vi "SBE45通讯参数 (子VI).vi"() -> (0 "错误输出":errorcluster, 1 "Salinity":string, 2 "Conductivity":string, 3 "Temperature":string)   [LabVIEW 2016]
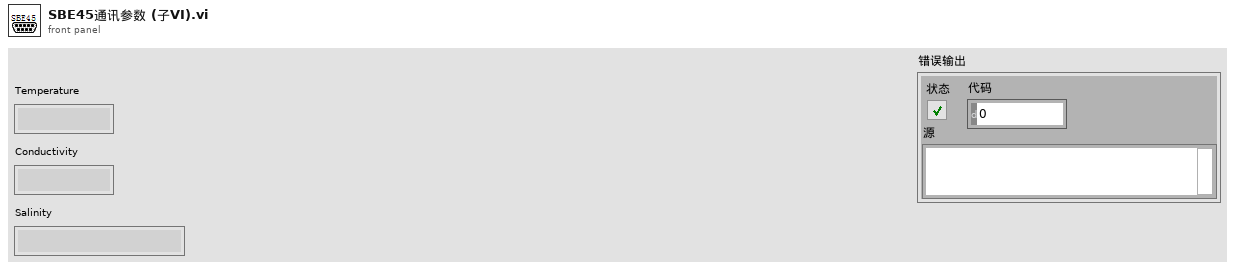
[diagram p1: front panel]
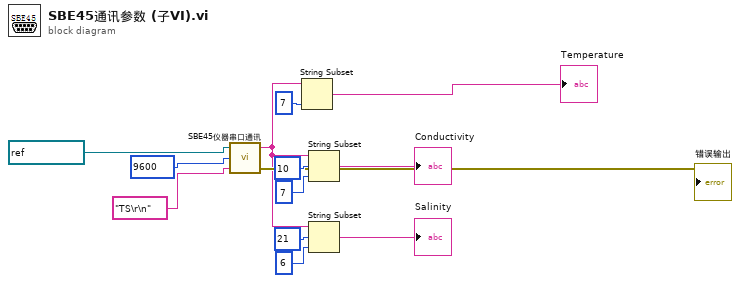
[diagram p0: block diagram]
diagram:
  n1 = call "SBE45仪器串口通讯.vi"("输入指令"="TS\r\n", "baud rate (9600)"=u32 9600, "VISA resource name"=refnum<visa-resource-name> "COM7") -> ("错误输出"=→"错误输出":errorcluster, "子字符串;substring"=w1:string)  [unwired: 1 out]
  n2 = String Subset(string=w1, length (rest)=7 ("长度（剩余）")) -> (substring=→"Temperature":string)  [unwired: 1 in]
  n3 = String Subset(string=w1, offset (0)=10 ("偏移量(0)"), length (rest)=7 ("长度（剩余）")) -> (substring=→"Conductivity":string)
  n4 = String Subset(string=w1, offset (0)=21 ("偏移量(0)"), length (rest)=6 ("长度（剩余）")) -> (substring=→"Salinity":string)
